vi "Set parameters.vi"(8 "error in (no error)":errorcluster caption="entrée d'erreur (pas d'erreur)", 11 "DLOwis en entrée":refnum<class "DLOwis.lvclass">) -> (0 "error out":errorcluster caption="sortie d'erreur", 3 "DLOwis en sortie":refnum<class "DLOwis.lvclass">)   [LabVIEW 2018, in "DLOwis.lvclass"]
uses:
  DLOwis.lvclass
  DelayLine.lvclass
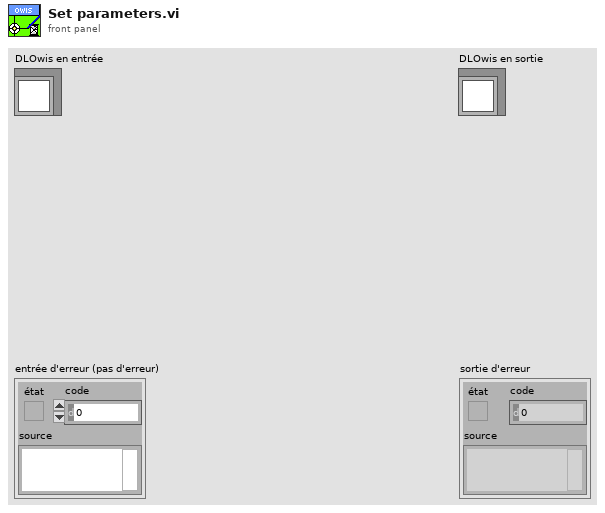
[diagram p1: front panel]
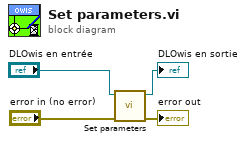
[diagram p0: block diagram]
diagram:
  n1 = call-parent "Set parameters.vi"("error in (no error)"="error in (no error)", "DelayLine en entrée"="DLOwis en entrée") -> ("error out"=→"error out":errorcluster, "DelayLine en sortie"=→"DLOwis en sortie":refnum<class "DLOwis.lvclass">)  [unwired: 8 in]
